vi "ExcitationParameters.vi"(7 "outputSensitivity":dbl, 8 "error in":errorcluster, 9 "excitationParameters":T2, 10 "ioFreqHz":u32, 11 "FPGA VI Reference In":T1) -> (0 "error out":errorcluster, 2 "WaveSize":i32, 3 "FPGA VI Reference Out":T1, 4 "Excitation":dbl[](array[numeric]))   [LabVIEW 2016]
uses:
  controls/FPGAVIreferenceTypeDef.ctl
  controls/Enum.ctl
  <vilib>/rvi/errors/niLvFpgaAdjustHostInterfaceError.vi
  <vilib>/Utility/error.llb/Error Cluster From Error Code.vi
  <vilib>/rvi/interface/nirviReadWriteControl/nirviReadWriteControl.xnode
  FPGA Bitfiles/qnmController797_usbRIO_controllerFPGAmu.lvbitx
  <vilib>/measure/NI_MABase.lvlib
  NiFpgaLv.dll
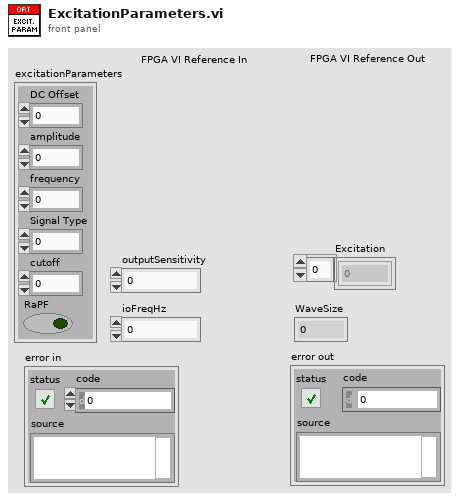
[diagram p1: front panel]
types:
  T1 = typedef "FPGAVIreferenceTypeDef.ctl" = refnum<k20>
  T2 = cluster{"DC Offset":dbl, "amplitude":dbl, "frequency":dbl, "Signal Type":u16, "cutoff":dbl, "RaPF":bool}
  T3 = typedef "Enum.ctl" = enum16{"Init", "Read", "Write"}
  T4 = cluster{"maxLoc":u16, "threshold":i16, "fitHardPtLimit":u16}
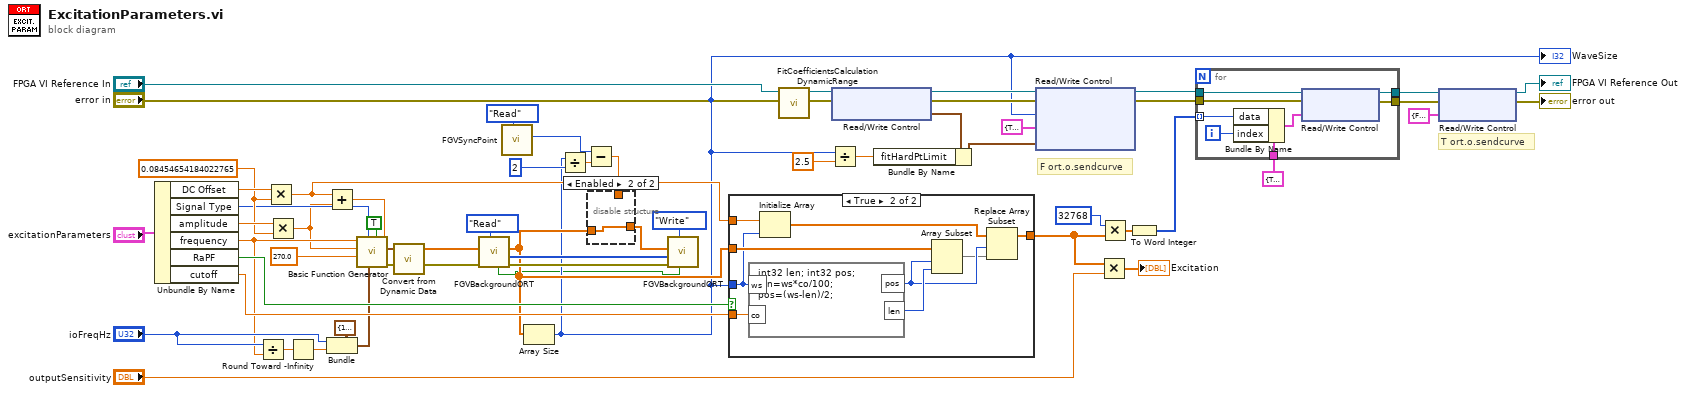
[diagram p0: block diagram]
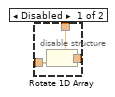
[diagram p2: hidden frame]
diagram:
  w37 = 0.08454654184022765 ("y")
  # "F ort.o.sendcurve"
  # "T ort.o.sendcurve"
  n1 = Unbundle By Name("excitationParameters") -> ("DC Offset"=w56:dbl, "Signal Type"=w13:u16, "amplitude"=w47:dbl, "frequency"=w12:dbl, "RaPF"=w54:bool, "cutoff"=w55:dbl)
  n2 = Divide(x="ioFreqHz", y=w12) -> (x/y=w40:dbl)
  n3 = Multiply(x=w56, y=w37) -> (x*y=w57:dbl)
  n4 = Multiply(x=w47, y=w37) -> (x*y=w11:dbl)
  n5 = Round Toward -Infinity(1:w40) -> (0:w39:dbl)
  n6 = Add(x=w57, y=w11) -> (x+y=w15:dbl)
  n7 = Bundle(cluster=cluster{"Fs":dbl, "#s":dbl} {"Fs"=1000000.0, "#s"=99.0} ("sampling info"), "Fs"="ioFreqHz", "#s"=w39) -> (w10:cluster{"Fs":dbl, "#s":dbl})
  n8 = call <vilib>:"Basic Function Generator.vi"("offset"=w15, "reset signal"=TRUE, "sampling info"=w10, "signal type"=w13, "phase"=270.0, "amplitude"=w11, "frequency"=w12) -> ("error out"=w33:errorcluster, "signal out"=w44:waveform(dbl))  [unwired: 2 in, 1 out]
  n9 = call "Convert from Dynamic Data"("Dynamic Data Type"=w44) -> ("Array"=w7:dbl[])  [unwired: 3 in]
  n10 = call "FGVBackgroundORT.vi"("Enum"=Enum."Read", "error in"=w33) -> ("error out"=w32:errorcluster, "arrayOut"=w31:i16[], "Corrected...Out"=w1:bool)  [unwired: 5 in, 2 out]
  n11 = call "FGVSyncPoint.vi"("Enum"=Enum."Read") -> ("SyncPointOut"=w6:u16)  [unwired: 9 in, 1 out]
  n12 = Array Size(array=w7) -> (size(s)=w2:i32)
  "WaveSize" <- w2
  n13 = Divide(x=w2, y=2 ("x")) -> (x/y=w4:dbl)
  n14 = Subtract(x=w6, y=w4) -> (x-y=w5:dbl)
  n15 = disable-structure shown="Enabled" {
    disable-tunnel: [w60 w61] -> w8
    disable-tunnel: w7 -> [w59 w61]
    disable-tunnel: w5 -> [w58 _]
    frame Disabled {
      n16 = Rotate 1D Array(1:w59, 2:w58) -> (0:w60:dbl[])
    }
    frame Enabled {
    }
  }
  n17 = call "FGVBackgroundORT.vi"("Corrected...In"=w1, "Enum"=Enum."Write", "error in"=w32, "arrayIn"=w31, "Wave In"=w8) -> ()  [unwired: 2 in, 5 out]
  n18 = case shown="True" w54 {
    tunnel: [w62 w63] -> w53
    tunnel: w7 -> [w62 w69]
    tunnel: w2 -> [_ w68]
    tunnel: w57 -> [_ w71]
    tunnel: w55 -> [_ w67]
    frame False {
    }
    frame True {
      n19 = formula code="int32 len; int32 pos;\nlen=ws*co/100;\npos=(ws-len)/2;"("ws"=w68, "co"=w67) -> ("len"=w66:i32, "pos"=w65:i32)
      n20 = Initialize Array(w71, w68) -> (w70:dbl[])
      n21 = Array Subset(array=w69, index=w65, length=w66) -> (w64:dbl[])
      n22 = Replace Array Subset(array=w70, new element=w64, index=w65) -> (w63:dbl[])
    }
  }
  n23 = call "FitCoefficientsCalculationDynamicRange.vi"("ArraySize"=w2, "FPGA VI Reference In"="FPGA VI Reference In") -> ("FPGA VI Reference Out"=w30:T1)  [unwired: 9 in]
  n24 = Divide(x=w2, y=2.5) -> (x/y=w49:dbl)
  n25 = xnode "Read/Write Control"("FPGA VI Reference In"=w30, "error in"="error in") -> ("FPGA VI Reference Out"=w18:T1, "error out"=w17:errorcluster, "ort.fit.p.params"=w28:T4)
  n26 = Bundle By Name(cluster=w28, "fitHardPtLimit"=w49) -> (w21:T4)
  n27 = xnode "Read/Write Control"("FPGA VI Reference In"=w18, "error in"=w17, "ort.p.waveSize"=w2, "aio.m.drive"=cluster{"write":bool, "data":i16, "index":u16} {"write"=TRUE, "data"=0, "index"=0} ("outWaveWrite"), "ort.fit.p.params"=w21) -> ("FPGA VI Reference Out"=w20:T1, "error out"=w19:errorcluster)
  n28 = Multiply(x=w53, y="outputSensitivity") -> (x*y=→"Excitation":dbl[])
  n29 = Multiply(x=32768, y=w53) -> (x*y=w52:dbl[])
  n30 = To Word Integer(number=w52) -> (16bit integer=w45:i16[])
  n31 = for {
    tunnel: w45 -> [w78] mode=indexing
    tunnel: w20 -> [w77]
    tunnel: [w75] -> w25
    tunnel: w19 -> [w74]
    tunnel: [w73] -> w26
    tunnel: cluster{"write":bool, "data":i16, "index":u16} {"write"=TRUE, "data"=0, "index"=0} ("outWaveWrite") -> [w72]
    i -> [w79]
    n32 = Bundle By Name(cluster=w72, "data"=w78, "index"=w79) -> (w76:cluster{"write":bool, "data":i16, "index":u16})
    n33 = xnode "Read/Write Control"("FPGA VI Reference In"=w77, "error in"=w74, "aio.m.drive"=w76) -> ("FPGA VI Reference Out"=w75:T1, "error out"=w73:errorcluster)
  }
  n34 = xnode "Read/Write Control"("FPGA VI Reference In"=w25, "error in"=w26, "aio.m.drive"=cluster{"write":bool, "data":i16, "index":u16} {"write"=FALSE, "data"=0, "index"=0} ("outWaveWrite")) -> ("FPGA VI Reference Out"=→"FPGA VI Reference Out":T1, "error out"=→"error out":errorcluster)
